vi "Read Sets pace.vi"(8 "error in (no error)":errorcluster, 11 "Mag Lab Result in":refnum<class "Mag Lab Result.lvclass">) -> (0 "error out":errorcluster, 2 "Sets pace":bool, 3 "Mag Lab Result out":refnum<class "Mag Lab Result.lvclass">)   [LabVIEW 2015, in "Mag Lab Result.lvclass"]
uses:
  Mag Lab Result.lvclass
  Mag Lab Result.lvclass/Mag Lab Result.ctl
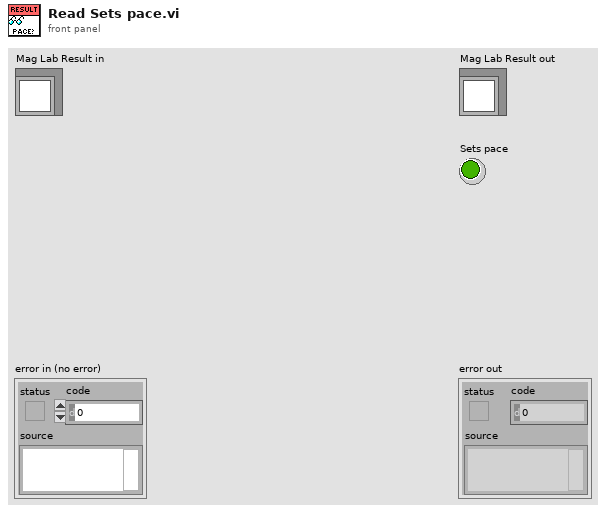
[diagram p1: front panel]
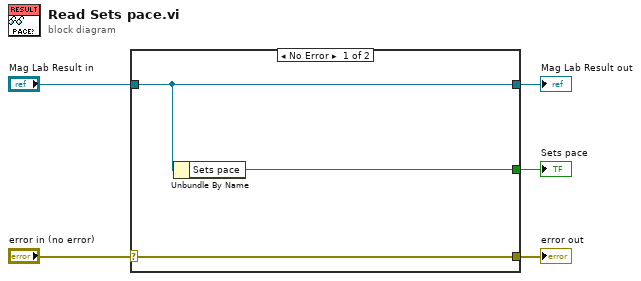
[diagram p0: block diagram]
diagram:
  n1 = case shown="No Error" "error in (no error)" {
    selector: "error in (no error)" -> [w8 w9]
    tunnel: [w8 w9] -> w4
    tunnel: [w7 w10] -> w2
    tunnel: "Mag Lab Result in" -> [w7 w10]
    tunnel: [w6 _] -> w1
    frame No Error {
      n2 = Unbundle By Name(w7) -> ("Sets pace"=w6:bool)
    }
    frame Error {
    }
  }
  "error out" <- w4
  "Mag Lab Result out" <- w2
  "Sets pace" <- w1
